vi "Move Fwd PID.vi"(4 "Loop Timer":i32=20, 5 "Gains":T1={"proportional gain (Kc)"=1.0, "integral time (Ti, min)"=0.01, "derivative time (Td, min)"=0.0} {"derivative time (Td, min)" format="%.3f"; "integral time (Ti, min)" format="%.3f"; "proportional gain (Kc)" format="%.3f"}, 7 "Range":cluster{"output high":dbl, "output low":dbl}={"output high"=1.0, "output low"=0.0} {"output low" format="%.2f"; "output high" format="%.2f"}, 8 "Precision":dbl=0.5 format="%#_13g", 9 "Time to stop":i32=300, 10 "Encoder Count":dbl, 11 "Distance":dbl) -> (0 "Output":dbl, 3 "Finished?":bool)   [LabVIEW 2017]
panel:
  in  "Soft start":dbl=1.0
  # "Time to stop - Tempo que o encoder deve retornar um valor dentro do range da precision para a função considerar que o sistema está parado.\n\nDistance - Setpoint em unidades do encoder.\n\nLoop Timer - Tempo de iteração do loop em que a função está.\n\nPrecision - Range que a função considera \"close enough\" ao setpoint.\n\nEncoder Count - Valor atual do encoder.\n\nRate limit - Limite de aceleração/desaceleração do sistema.\n\nGains - Ganhos do PID.\n\nRange - limite superior e inferior do PID.\n\nSoft Start - constante que aumenta ou diminui o tempo de aceleração no início do movimento"
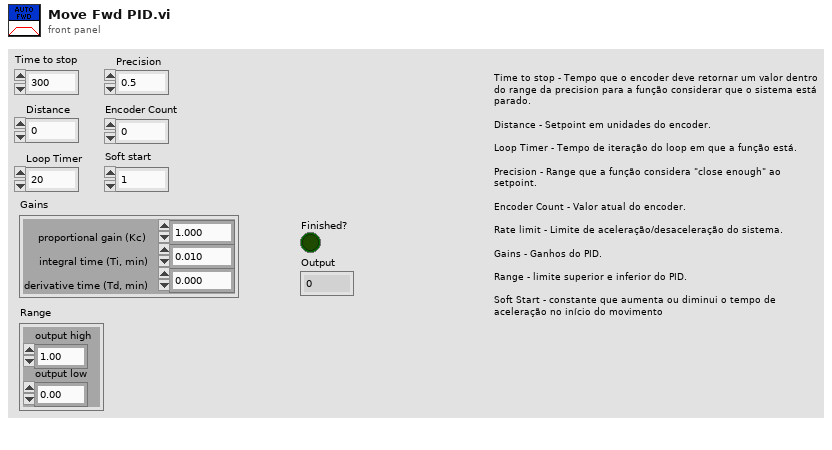
[diagram p1: front panel]
types:
  T1 = cluster{"proportional gain (Kc)":dbl, "integral time (Ti, min)":dbl, "derivative time (Td, min)":dbl}
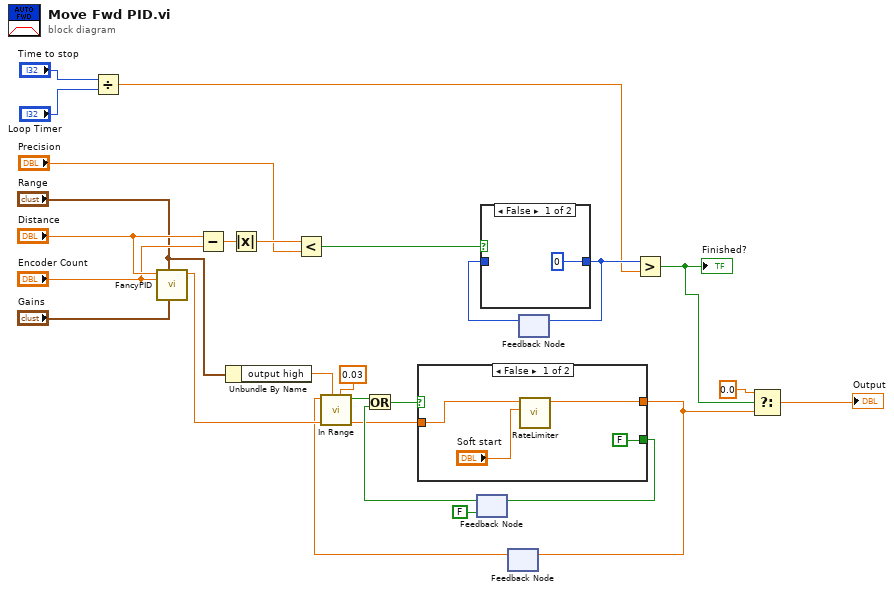
[diagram p0: block diagram]
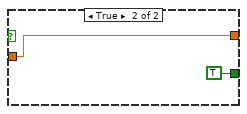
[diagram p2: hidden frame]
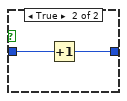
[diagram p3: hidden frame]
diagram:
  n1 = Divide(x="Time to stop", y="Loop Timer") -> (x/y=w20:dbl)
  n2 = call "FancyPID.vi"("Gains"="Gains", "Range"="Range", "Process variable"="Encoder Count", "Setpoint"="Distance") -> ("output"=w6:dbl)  [unwired: 7 in]
  n3 = Subtract(x="Distance", y="Encoder Count") -> (x-y=w19:dbl)
  n4 = Unbundle By Name("Range") -> ("output high"=w13:dbl)
  n5 = Absolute Value(x=w19) -> (abs(x)=w25:dbl)
  n6 = Less?(x=w25, y="Precision") -> (x < y?=w23:bool)
  n7 = feedback #1(FALSE) -> (w8:bool)
  n8 = feedback #2() -> (w5:dbl)  [unwired: 1 in]
  n9 = call "In Range.vi"("Range"=0.03, "Setpoint"=w13, "Value"=w5) -> ("in range?"=w11:bool)  [unwired: 8 in]
  n10 = Or(x=w11, y=w8) -> (x .or. y?=w10:bool)
  n11 = case shown="False" w10 {
    tunnel: [w30 w31] -> w3
    tunnel: w6 -> [w29 w31]
    tunnel: [FALSE TRUE] -> w9
    frame False {
      n12 = call "RateLimiter.vi"("Max dx/dt"="Soft start", "Input"=w29) -> ("Output"=w30:dbl)  [unwired: 9 in]
    }
    frame True {
    }
  }
  n13 = feedback-in #1(w9) -> ()
  n14 = feedback-in #2(w3) -> ()
  n15 = feedback #3() -> (w22:i32)  [unwired: 1 in]
  n16 = case shown="False" w23 {
    tunnel: [0 w35] -> w21
    tunnel: w22 -> [_ w34]
    frame False {
    }
    frame True {
      n17 = Increment(x=w34) -> (x+1=w35:i32)
    }
  }
  n18 = feedback-in #3(w21) -> ()
  n19 = Greater?(x=w21, y=w20) -> (0:w1:bool)
  "Finished?" <- w1
  n20 = Select(t=0.0, s=w1, f=w3) -> (s? t:f=→"Output":dbl)
